vi "RT Error Handler - DAQ Control.vi"(8 "error in (no error)":errorcluster caption="错误输入（无错误）", 11 "Message Queue":refnum<queue> caption="消息队列") -> (2 "Enqueued Error?":bool caption="错误入队列？", 3 "dup Message Queue":refnum<queue> caption="消息队列副本")   [LabVIEW 2013]
uses:
  support/Message Queue/Message Cluster.ctl
  controls/Error Type.ctl
  support/Message Queue/Message Queue.lvlib
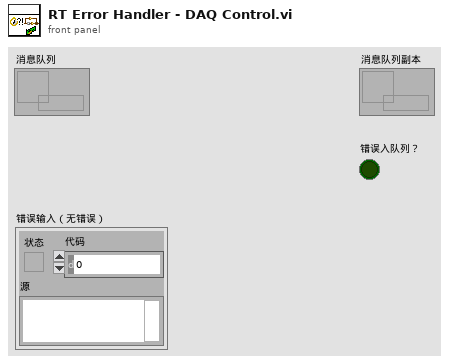
[diagram p1: front panel]
types:
  T1 = typedef "Error Type.ctl" = enum16{"Log-Only Error", "Non-Critical Error", "Critical Error"}
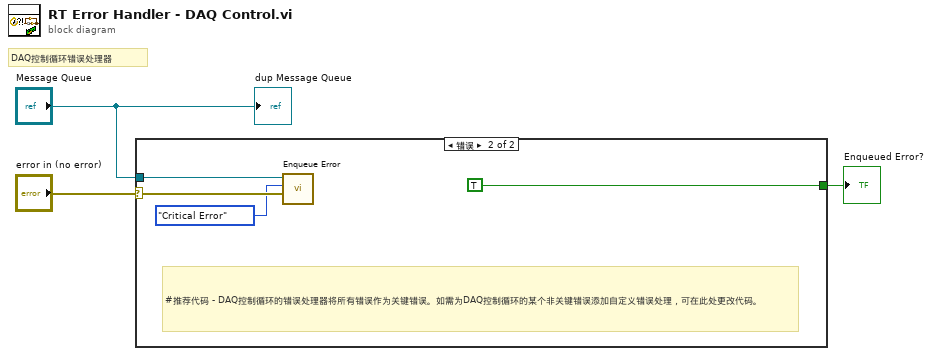
[diagram p0: block diagram]
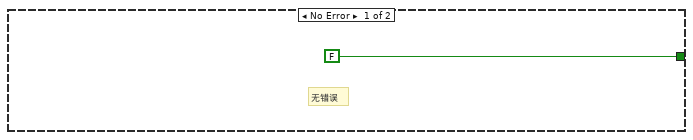
[diagram p2: hidden frame]
diagram:
  # "DAQ控制循环错误处理器"
  n1 = case shown="错误" "error in (no error)" {
    selector: "error in (no error)" -> [_ w7]
    tunnel: "Message Queue" -> [_ w8]
    tunnel: [FALSE ("Enqueued Error?") TRUE ("Enqueued Error?")] -> w2
    frame No Error {
      # "无错误"
    }
    frame Error {
      # "#推荐代码 - DAQ控制循环的错误处理器将所有错误作为关键错误。如需为DAQ控制循环的某个非关键错误添加自定义错误处理，可在此处更改代码。"
      n2 = call "Enqueue Error.vi"("error to process"=w7, "Error Type (Non-Critical)"=Error_Type."Critical Error", "Message Queue"=w8) -> ()  [unwired: 9 in]
    }
  }
  "Enqueued Error?" <- w2
  "dup Message Queue" <- "Message Queue"
